vi "Set RFM Interrupt Enabled States.vi"(8 "error in (no error)":errorcluster, 10 "Interrupt Enables":T1, 11 "GE 5565PIORC in":refnum<class "GE 5565PIORC.lvclass">) -> (0 "error out":errorcluster, 3 "GE 5565PIORC out":refnum<class "GE 5565PIORC.lvclass">)   [LabVIEW 2016, in "GE 5565PIORC.lvclass"]
uses:
  GE 5565PIORC.lvclass
  Controls/Interrupt Enables.ctl
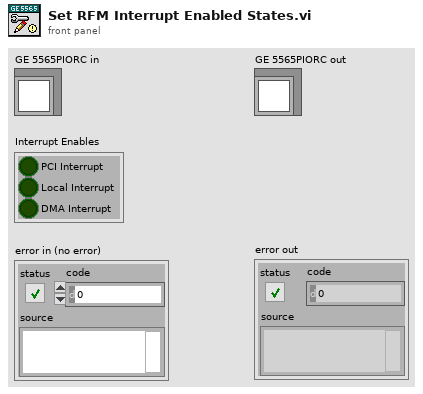
[diagram p1: front panel]
types:
  T1 = typedef "GE 5565PIORC.lvclass/Interrupt Enables.ctl" = cluster{"PCI Interrupt":bool, "Local Interrupt":bool, "DMA Interrupt":bool}
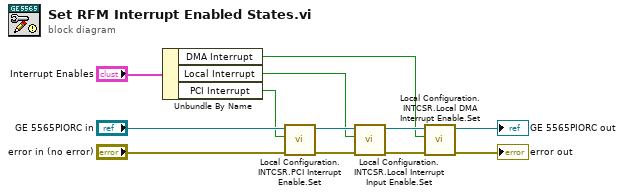
[diagram p0: block diagram]
diagram:
  n1 = Unbundle By Name("Interrupt Enables") -> ("DMA Interrupt"=w1:bool, "Local Interrupt"=w2:bool, "PCI Interrupt"=w3:bool)
  n2 = call "Local Configuration.INTCSR.PCI Interrupt Enable.Set.vi"("error in (no error)"="error in (no error)", "Enable PCI Interrupt?"=w3, "GE 5565PIORC"="GE 5565PIORC in") -> ("error out"=w6:errorcluster, "GE 5565PIORC out"=w9:refnum<class "GE 5565PIORC.lvclass">)  [unwired: 7 in]
  n3 = call "Local Configuration.INTCSR.Local Interrupt Input Enable.Set.vi"("error in (no error)"=w6, "Enable Local Interrupt Input?"=w2, "GE 5565PIORC"=w9) -> ("error out"=w5:errorcluster, "GE 5565PIORC out"=w8:refnum<class "GE 5565PIORC.lvclass">)  [unwired: 7 in]
  n4 = call "Local Configuration.INTCSR.Local DMA Interrupt Enable.Set.vi"("error in (no error)"=w5, "Enable Local DMA Interrupt?"=w1, "GE 5565PIORC"=w8) -> ("error out"=→"error out":errorcluster, "GE 5565PIORC out"=→"GE 5565PIORC out":refnum<class "GE 5565PIORC.lvclass">)  [unwired: 7 in]
